vi "全局变量.vi"() -> ()   [LabVIEW 2011]
panel:
  out "Counter":i32
  in  "Flag":bool
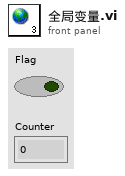
[diagram p1: front panel]
diagram:
